vi "Get Templates List.vi"(8 "Error In":errorcluster, 11 "Folder Path":path) -> (0 "Error Out":errorcluster, 3 "Templates List (Paths)":path[](array[path]))   [LabVIEW 2013, in "Scripter.lvlib"]
uses:
  Scripter.lvlib
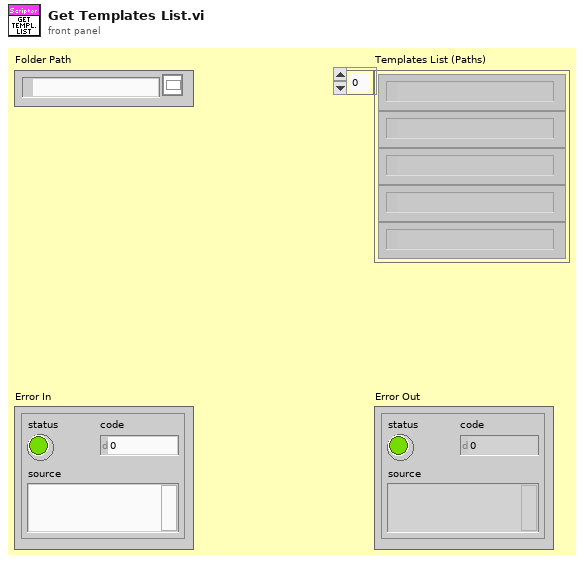
[diagram p1: front panel]
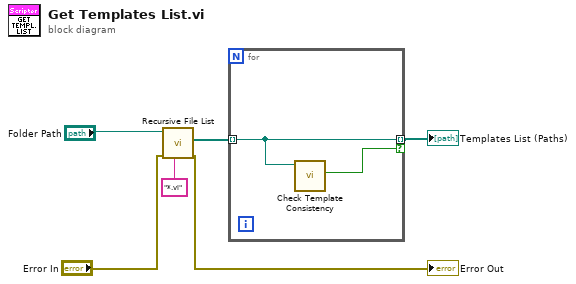
[diagram p0: block diagram]
diagram:
  n1 = call <vilib>:"Recursive File List.vi"("pattern"="*.vi", "error in (no error)"="Error In", "Folder Path"="Folder Path") -> ("error out"=→"Error Out":errorcluster, "All Files in Dir"=w4:path[])  [unwired: 4 in, 3 out]
  n2 = for {
    tunnel: w4 -> [w8] mode=indexing
    tunnel: [w8] -> w3 mode=indexing if=w7
    n3 = call "Check Template Consistency.vi"("Template Method Path"=w8) -> ("Template is OK?"=w7:bool)  [unwired: 10 in]
  }
  "Templates List (Paths)" <- w3
